vi "Sub_Online_FEA_Sample_Nodes.vi"(8 "include extremes":bool, 9 "Modeling Parameters":T1, 10 "FEA Nodes":i32[](array[numeric]), 11 "Initial Pin Location":i32) -> (1 "Unique Samples":i32[](array[numeric]), 2 "Sample PDF":dbl[](array[numeric]), 3 "Standard Deviation":dbl)   [LabVIEW 2021]
uses:
  bb61caf6-2445-4ad4-a19b-d78b508e9aa3.vi
  b80c990e-e254-4647-8afe-47c3290e6feb.vi
  <vilib>/gmath/statdist.llb/Normal PDF.vi
  <vilib>/Comparison/Less/Less Functor/Less Functor.lvclass
  <vilib>/gmath/NI_Gmath.lvlib
panel:
  out "Waveform Graph":dbl[](graph)
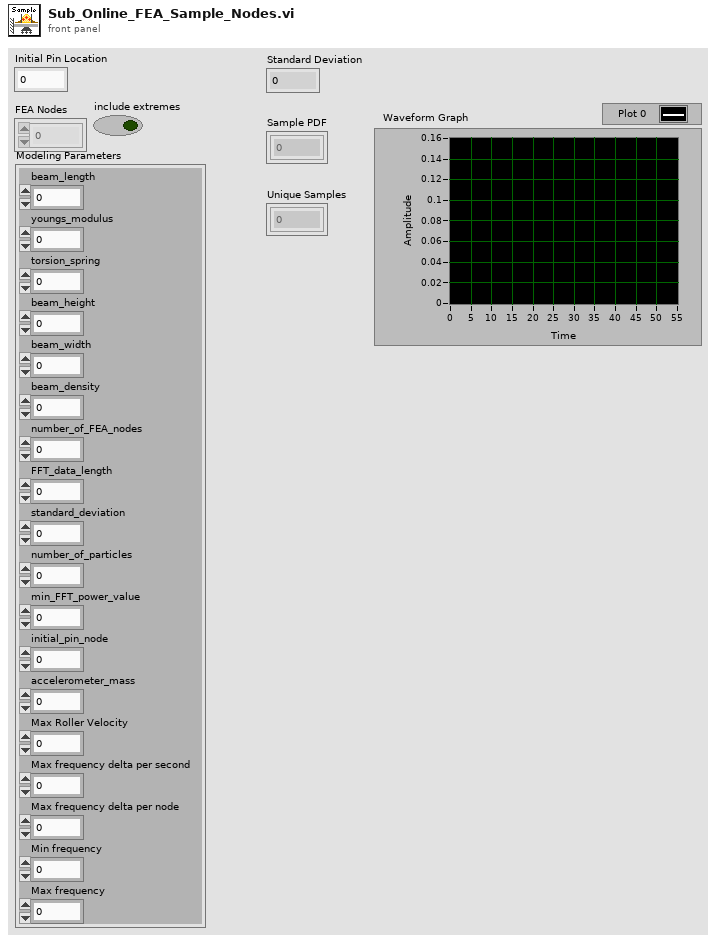
[diagram p1: front panel]
types:
  T1 = cluster{"beam_length":dbl, "youngs_modulus":dbl, "torsion_spring":dbl, "beam_height":dbl, "beam_width":dbl, "beam_density":dbl, "number_of_FEA_nodes":i32, "FFT_data_length":i32, "standard_deviation":dbl, "number_of_particles":i32, "min_FFT_power_value":dbl, "initial_pin_node":i32, "accelerometer_mass":dbl, "Max Roller Velocity":dbl, "Max frequency delta per second":dbl, "Max frequency delta per node":dbl, "Min frequency":dbl, "Max frequency":dbl}
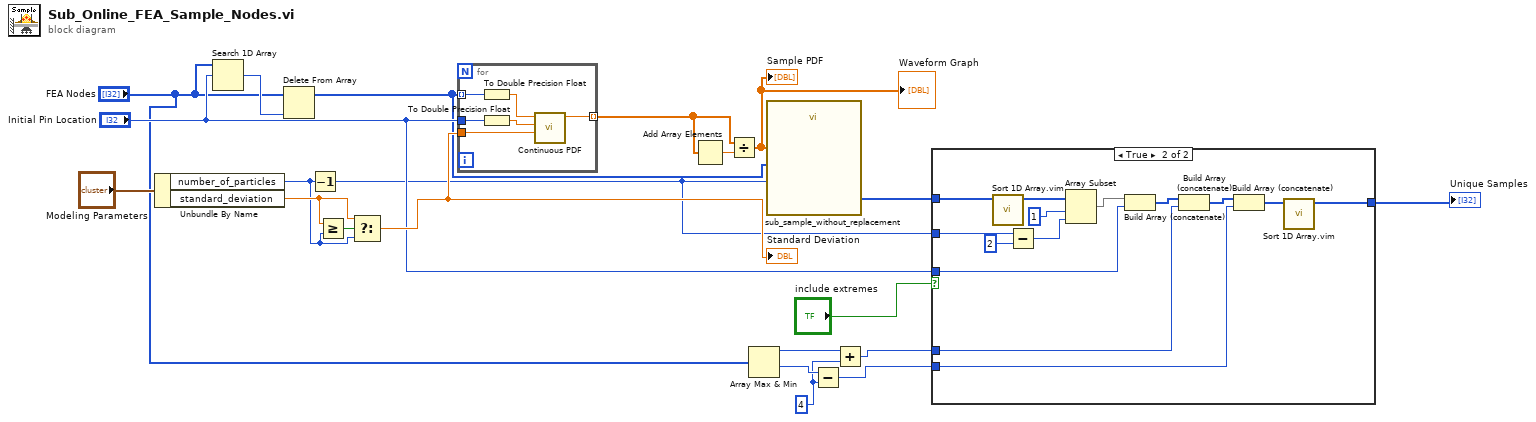
[diagram p0: block diagram]
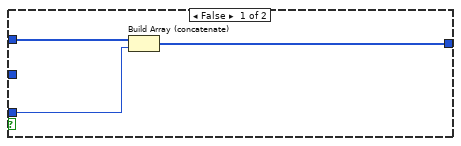
[diagram p2: hidden frame]
diagram:
  w1 = 4 ("y")
  n1 = Unbundle By Name("Modeling Parameters") -> ("number_of_particles"=w16:i32, "standard_deviation"=w18:dbl)
  n2 = Search 1D Array(1D array="FEA Nodes", element="Initial Pin Location") -> (index of element=w10:i32)  [unwired: 1 in]
  n3 = Delete From Array(array="FEA Nodes", index=w10) -> (array with subset deleted=w7:i32[])  [unwired: 1 in, 1 out]
  n4 = Decrement(x=w16) -> (x-1=w9:i32)
  n5 = Greater Or Equal?(x=w18, y=w16) -> (x >= y?=w19:bool)
  n6 = Select(t=w18, s=w19, f=w16) -> (s? t:f=w17:dbl)
  "Standard Deviation" <- w17
  n7 = for {
    tunnel: w7 -> [w24] mode=indexing
    tunnel: [w27] -> w20 mode=indexing
    tunnel: "Initial Pin Location" -> [w23]
    tunnel: w17 -> [w26]
    n8 = To Double Precision Float(number=w24) -> (double precision float=w25:dbl)
    n9 = To Double Precision Float(number=w23) -> (double precision float=w22:dbl)
    n10 = call-poly <vilib>:"Continuous PDF.vi"("std"=w26, "mean"=w22, "x"=w25) -> ("pdf(x)"=w27:dbl)  [unwired: 7 in, 1 out]
  }
  n11 = Add Array Elements(numeric array=w20) -> (sum=w21:dbl)
  n12 = Divide(x=w20, y=w21) -> (x/y=w15:dbl[])
  "Sample PDF" <- w15
  "Waveform Graph" <- w15
  n13 = Array Max & Min(array="FEA Nodes") -> (max value=w4:i32, min value=w5:i32)  [unwired: 2 out]
  n14 = call "sub_sample_without_replacement.vi"("number of unique samples"=w9, "probability"=w15, "List"=w7) -> ("unique samples"=w13:i32[])  [unwired: 6 in, 2 out]
  n15 = Subtract(x=w5, y=w1) -> (x-y=w2:i32)
  n16 = Add(x=w4, y=w1) -> (x+y=w3:i32)
  n17 = case shown="True" "include extremes" {
    tunnel: w13 -> [w30 w44]
    tunnel: [w28 w31] -> w12
    tunnel: "Initial Pin Location" -> [w29 w35]
    tunnel: w3 -> [_ w34]
    tunnel: w2 -> [_ w33]
    tunnel: w9 -> [_ w41]
    frame False {
      n18 = Build Array (concatenate)(w30, w29) -> (w28:i32[])
    }
    frame True {
      n19 = call "Sort 1D Array.vim"("unsorted array"=w44) -> ("sorted array"=w43:i32[])  [unwired: 10 in]
      n20 = Subtract(x=w41, y=2) -> (x-y=w40:i32)
      n21 = Array Subset(array=w43, index=1, length=w40) -> (w38:i32[])
      n22 = Build Array (concatenate)(w38, w35) -> (w37:i32[])
      n23 = Build Array (concatenate)(w37, w34) -> (w36:i32[])
      n24 = Build Array (concatenate)(w36, w33) -> (w32:i32[])
      n25 = call "Sort 1D Array.vim"("unsorted array"=w32) -> ("sorted array"=w31:i32[])  [unwired: 10 in]
    }
  }
  "Unique Samples" <- w12
